vi "RT - Count2Speed.vi"(8 "error in":errorcluster, 11 "RotaryMotorVelocityCounts/Interval":i16) -> (0 "error out":errorcluster, 3 "Velocity (RPM)":dbl)   [LabVIEW 2018]
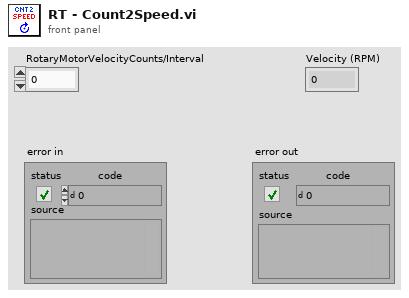
[diagram p1: front panel]
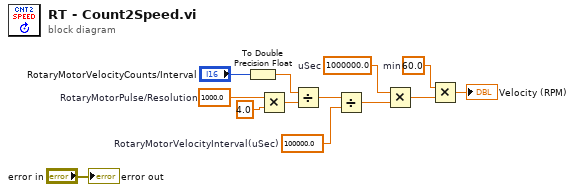
[diagram p0: block diagram]
diagram:
  w12 = 60.0  # min
  w10 = 1000000.0  # uSec
  w8 = 100000.0  # RotaryMotorVelocityInterval(uSec)
  w2 = 1000.0  # RotaryMotorPulse/Resolution
  n1 = To Double Precision Float(number="RotaryMotorVelocityCounts/Interval") -> (double precision float=w5:dbl)
  n2 = Multiply(x=w2, y=4.0) -> (x*y=w6:dbl)
  n3 = Divide(x=w5, y=w6) -> (x/y=w7:dbl)
  n4 = Divide(x=w7, y=w8) -> (x/y=w9:dbl)
  n5 = Multiply(x=w10, y=w9) -> (x*y=w11:dbl)
  n6 = Multiply(x=w12, y=w11) -> (x*y=→"Velocity (RPM)":dbl)
  "error out" <- "error in"
